vi "CalVision.vi"(10 "SerialPortIn":T1) -> (3 "SerialPortOut":T1)   [LabVIEW 2017, in "VisionHW.lvlib"]
uses:
  VisionHW.lvlib
  <vilib>/Rock Robotics/WPI/SerialPort/WPI_SerialPortRef.ctl
panel:
  out "Command":string
  in  "V Range":cluster{dbl, dbl}(slide) scale=0.0..255.0
  in  "S Range":cluster{dbl, dbl}(slide) scale=0.0..255.0
  in  "H Range":cluster{dbl, dbl}(slide) scale=0.0..255.0
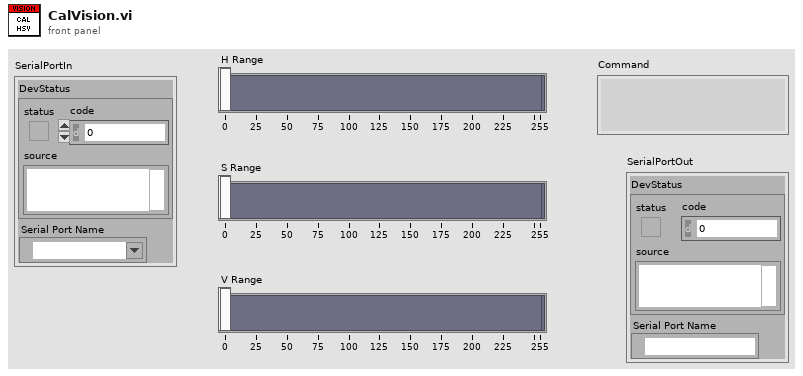
[diagram p1: front panel]
types:
  T1 = typedef "WPI_SerialPortRef.ctl" = cluster{"DevStatus":errorcluster, "Serial Port Name":refnum<visa-resource-name>}
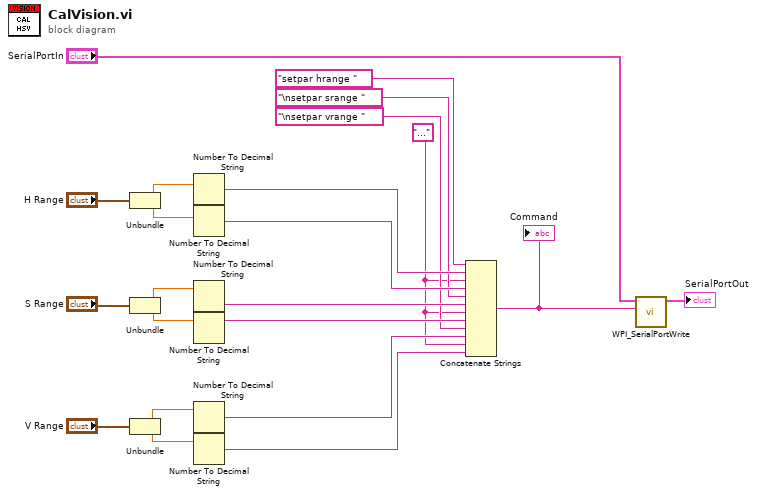
[diagram p0: block diagram]
diagram:
  w5 = "..." ("string")
  n1 = Unbundle("H Range") -> (w21:dbl, w18:dbl)
  n2 = Unbundle("S Range") -> (w14:dbl, w13:dbl)
  n3 = Unbundle("V Range") -> (w12:dbl, w11:dbl)
  n4 = Number To Decimal String(number=w21) -> (decimal integer string=w19:string)  [unwired: 1 in]
  n5 = Number To Decimal String(number=w18) -> (decimal integer string=w17:string)  [unwired: 1 in]
  n6 = Number To Decimal String(number=w14) -> (decimal integer string=w9:string)  [unwired: 1 in]
  n7 = Number To Decimal String(number=w13) -> (decimal integer string=w8:string)  [unwired: 1 in]
  n8 = Number To Decimal String(number=w12) -> (decimal integer string=w6:string)  [unwired: 1 in]
  n9 = Number To Decimal String(number=w11) -> (decimal integer string=w4:string)  [unwired: 1 in]
  n10 = Concatenate Strings("setpar hrange " ("string"), w19, w5, w17, "\nsetpar srange " ("string"), w9, w5, w8, "\nsetpar vrange " ("string"), w6, w5, w4) -> (w2:string)
  "Command" <- w2
  n11 = call <vilib>:"WPI_SerialPortWrite.vi"("Buffer"=w2, "SerialPortRef"="SerialPortIn") -> ("SerialPortRef"=→"SerialPortOut":T1)  [unwired: 7 in, 2 out]
